vi "测试-探头模板-有线版.vi"() -> ()   [LabVIEW 2016]
panel:
  in  "报警状态":enum16{"正常", "一级报警", "二级报警", "累积报警"}(ring)=enum."一级报警"
  in  "枚举":enum16{"2~8模板-有线版", "12模板-有线版"}(ring)
  in  "等待时间（毫秒）":u32=500
  in  "停止按钮":bool
  in  "限值":cluster{"限值1":dbl, "限值2":dbl}={"限值1"=1.0, "限值2"=100.0}
  in  "最低水平":dbl=0.15 format="%#_13g"
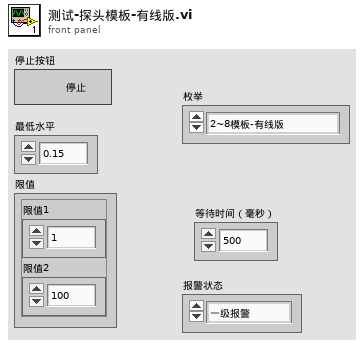
[diagram p1: front panel]
types:
  T1 = cluster{"启用状态？":bool, "测量值":cluster{"X":timestamp, "Y":dbl}, "限值簇":cluster{"限值1":dbl, "限值2":dbl}, "报警状态":enum16{"正常", "一级报警", "二级报警", "累积报警"}, "探头信息":string, "探头地址":i32, "累积剂量":cluster{"设备名称":string, "启用累积？":bool, "起始时间":timestamp, "累积剂量":dbl, "累积报警阈值":dbl}}
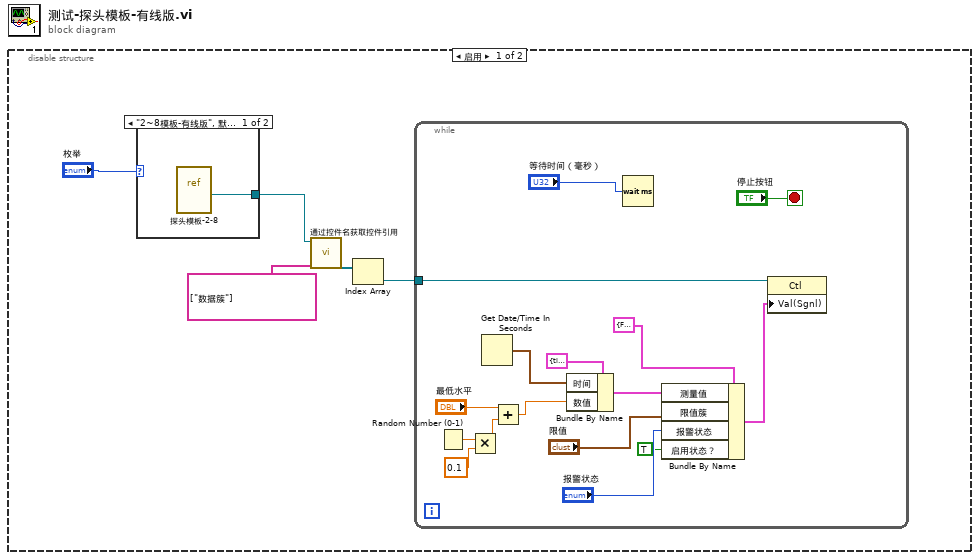
[diagram p0: block diagram]
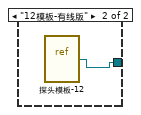
[diagram p2: hidden frame]
diagram:
  n1 = disable-structure shown="启用" {
    frame Enabled {
      n2 = case shown="\"2~8模板-有线版\", 默认" "枚举" {
        tunnel: [w6 w7] -> w5
        frame "2~8模板-有线版", Default {
          n3 = vi-ref "探头模板-2-8.vi"() -> (w6:refnum<vi>)
        }
        frame "12模板-有线版" {
          n4 = vi-ref "探头模板-12.vi"() -> (w7:refnum<vi>)
        }
      }
      n5 = call "通过控件名获取控件引用.vi"("控件名数组"=string[] ["数据簇"], "VI引用"=w5) -> ("控件引用输出"=w3:refnum<vi>[])  [unwired: 7 in, 2 out]
      n6 = Index Array(array=w3) -> (element=w2:refnum<vi>)  [unwired: 1 in]
      n7 = while {
        tunnel: w2 -> [w23]
        stop <- "停止按钮" stop-if-true
        n8 = Random Number (0-1)() -> (number: 0 to 1=w21:dbl)
        n9 = Multiply(x=w21, y=0.1) -> (x*y=w14:dbl)
        n10 = Get Date/Time In Seconds() -> (seconds since 1Jan1904=w20:timestamp)
        n11 = Add(x="最低水平", y=w14) -> (x+y=w19:dbl)
        n12 = Bundle By Name(cluster=cluster{"时间":timestamp, "数值":dbl} {"时间"=timestamp(0 s since 1904-01-01), "数值"=0.0} ("测量值"), "时间"=w20, "数值"=w19) -> (w12:cluster{"时间":timestamp, "数值":dbl})
        n13 = Wait (ms)(milliseconds to wait="等待时间（毫秒）") -> ()  [unwired: 1 out]
        n14 = Bundle By Name(cluster=T1 {"启用状态？"=FALSE, "测量值"={"X"=timestamp(0 s since 1904-01-01), "Y"=0.0}, "限值簇"={"限值1"=0.0, "限值2"=0.0}, "报警状态"=enum."正常", "探头信息"="", "探头地址"=0, "累积剂量"={"设备名称"="", "启用累积？"=FALSE, "起始时间"=timestamp(0 s since 1904-01-01), "累积剂量"=0.0, "累积报警阈值"=0.0}} ("新值"), "测量值"=w12, "限值簇"="限值", "报警状态"="报警状态", "启用状态？"=TRUE) -> (w17:T1)
        n15 = property class="Ctl"(reference=w23, "Val(Sgnl)"=w17) -> ()  [unwired: 1 in, 2 out]
      }
    }
    frame Disabled {
    }
  }
